vi "Data to Excel.vi"(6 "Hoje":string, 7 "Proxima":string, 8 "Error In":errorcluster, 9 "Control":enum16{"Get", "Set"}(ring), 10 "Patrim":string, 11 "Controle":string) -> (0 "Error Out":errorcluster, 1 "Patrim Out":string, 2 "Controle Out":string, 3 "Proxima Out":string, 4 "Hoje out":string)   [LabVIEW 2015]
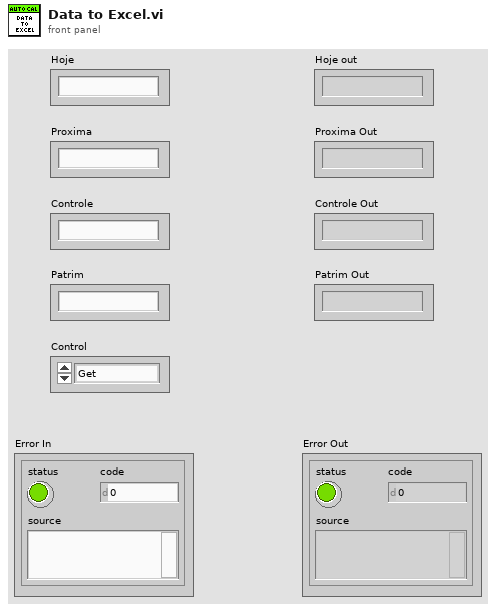
[diagram p1: front panel]
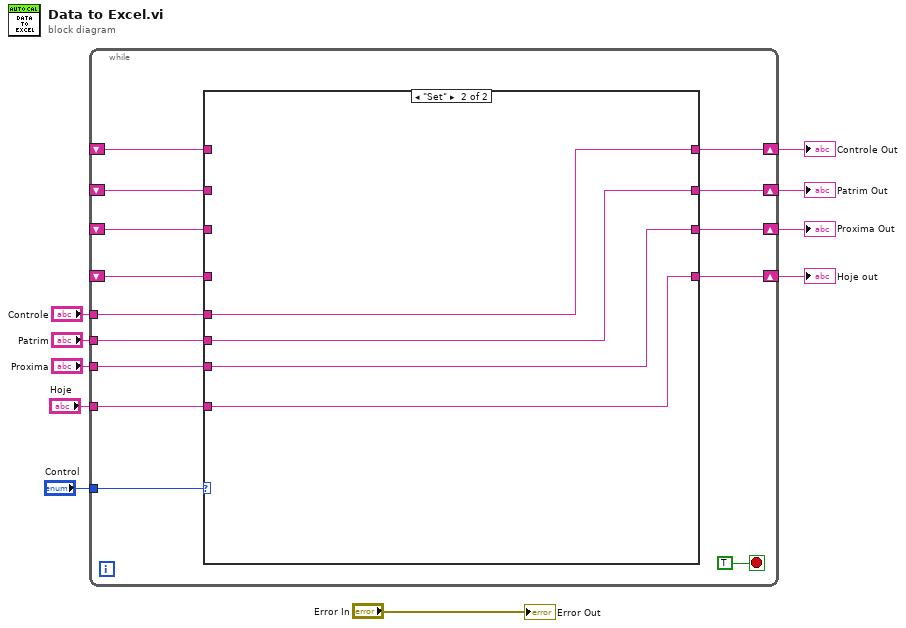
[diagram p0: block diagram]
diagram:
  n1 = while {
    tunnel: "Control" -> [w23]
    tunnel: "Controle" -> [w21]
    tunnel: "Patrim" -> [w20]
    tunnel: "Proxima" -> [w18]
    shift-right: [w22] -> w9
    shift-left: _ -> [w16]
    shift-right: [w19] -> w3
    shift-left: _ -> [w15]
    shift-right: [w17] -> w4
    shift-left: _ -> [w14]
    tunnel: "Hoje" -> [w13]
    shift-right: [w12] -> w1
    shift-left: _ -> [w11]
    stop <- TRUE stop-if-true
    n2 = case shown="\"Set\"" w23 {
      tunnel: [w28 w32] -> w22
      tunnel: w21 -> [_ w32]
      tunnel: w20 -> [_ w31]
      tunnel: [w27 w31] -> w19
      tunnel: w18 -> [_ w30]
      tunnel: [w26 w30] -> w17
      tunnel: w16 -> [w28 _]
      tunnel: w15 -> [w27 _]
      tunnel: w14 -> [w26 _]
      tunnel: w13 -> [_ w29]
      tunnel: [w25 w29] -> w12
      tunnel: w11 -> [w25 _]
      frame "Get", Default {
      }
      frame "Set" {
      }
    }
  }
  "Patrim Out" <- w3
  "Proxima Out" <- w4
  "Controle Out" <- w9
  "Hoje out" <- w1
  "Error Out" <- "Error In"
